vi "Create File.vi"(8 "error in (no error)":errorcluster, 10 "File Name Prefix":string) -> (0 "error out":errorcluster, 3 "refnum out":refnum<file>)   [LabVIEW 2015]
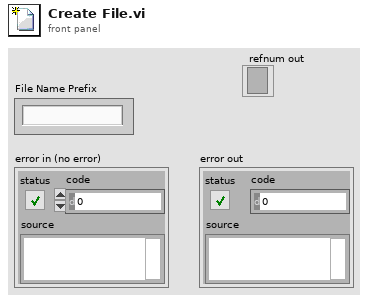
[diagram p1: front panel]
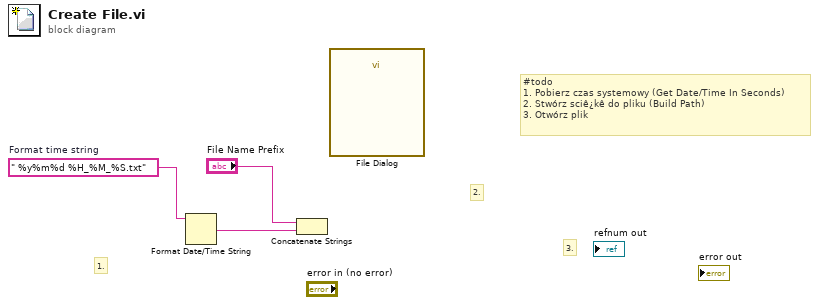
[diagram p0: block diagram]
diagram:
  w2 = " %y%m%d %H_%M_%S.txt"  # Format time string
  # "3."
  # "2."
  # "1."
  # "#todo\n1. Pobierz czas systemowy (Get Date/Time In Seconds)\n2. Stwórz sciê¿kê do pliku (Build Path)\n3. Otwórz plik"
  n1 = Format Date/Time String(time format string (%c)=w2) -> (date/time string=w3:string)  [unwired: 2 in]
  n2 = Concatenate Strings("File Name Prefix", w3) -> ()  [unwired: 1 out]
  n3 = call "File Dialog"() -> ()  [unwired: 12 in, 4 out]
